vi "Status Builder for ERD combo.vi"() -> ()   [LabVIEW 2016]
panel:
  out "Array":string[](array[string])
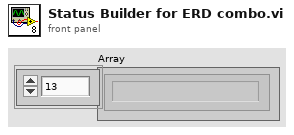
[diagram p1: front panel]
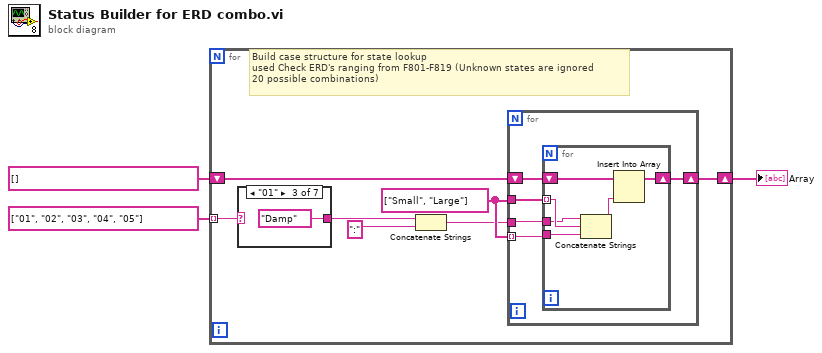
[diagram p0: block diagram]
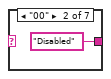
[diagram p3: hidden frame]
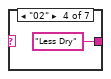
[diagram p4: hidden frame]
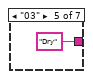
[diagram p5: hidden frame]
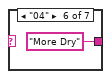
[diagram p6: hidden frame]
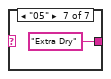
[diagram p7: hidden frame]
diagram:
  n1 = for {
    tunnel: string[] ["01", "02", "03", "04", "05"] -> [w10] mode=indexing
    shift-right: [w4] -> w1
    shift-left: string[] [] -> [w5]
    w9 = string[] ["Small", "Large"]
    # "Build case structure for state lookup \nused Check ERD's ranging from F801-F819 (Unknown states are ignored\n20 possible combinations)"
    n2 = case shown="\"01\"" w10 {
      selector: w10 -> [w22 _ _ _ _ _ _]
      tunnel: [w22 "Disabled" "Damp" "Less Dry" "Dry" "More Dry" "Extra Dry"] -> w8
      frame Default {
      }
      frame "00" {
      }
      frame "01" {
      }
      frame "02" {
      }
      frame "03" {
      }
      frame "04" {
      }
      frame "05" {
      }
    }
    n3 = Concatenate Strings(w8, ":" ("string")) -> (w6:string)
    n4 = for {
      tunnel: w9 -> [w11] mode=indexing
      tunnel: w9 -> [w15]
      tunnel: w6 -> [w12]
      shift-right: [w13] -> w4
      shift-left: w5 -> [w14]
      n5 = for {
        tunnel: w15 -> [w17] mode=indexing
        tunnel: w11 -> [w18]
        shift-right: [w19] -> w13
        shift-left: w14 -> [w21]
        tunnel: w12 -> [w16]
        n6 = Concatenate Strings(w16, w17, w18) -> (w20:string)
        n7 = Insert Into Array(array=w21, new element=w20) -> (w19:string[])  [unwired: 1 in]
      }
    }
  }
  "Array" <- w1
